vi "Command Drive Distance.vi"(6 "Timeout":dbl=2.0, 8 "Speed":dbl=0.7, 9 "Heading":dbl, 10 "Distance(Feet)":dbl=-8.0, 11 "Startup":bool) -> (0 "Angular":dbl, 1 "Reinit":bool, 2 "Linear":dbl, 3 "Completed":bool=TRUE)   [LabVIEW 2019]
uses:
  Subsystems/Sensing/Sensor_Values.vi
  Auto Utilities/Command_Execution_State.ctl
panel:
  in  "Angle_Threshold":dbl=5.0
  in  "Agressive Turn P":dbl=0.2
  in  "Turn I":dbl=0.0001
  in  "Turn D":dbl=0.005
  out "Turning":cluster{"Heading":dbl, "Drive_IMU":dbl}(graph)={"Heading"=0.0, "Drive_IMU"=0.3076171875}
  in  "Normal Turn P":dbl=0.03
  in  "Distance Gain":dbl=0.01
  # "Alpha .06"
  # "Beta .1"
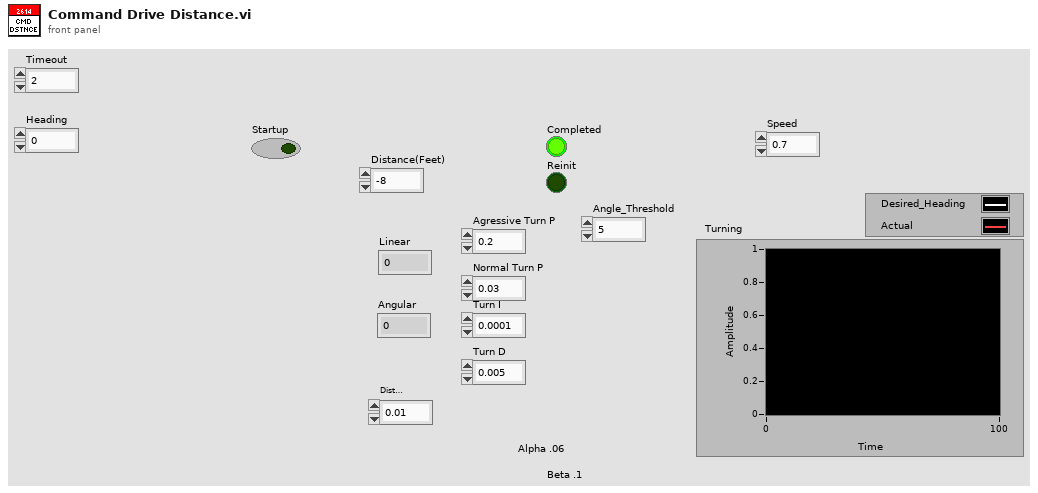
[diagram p1: front panel]
types:
  T1 = typedef "Command_Execution_State.ctl" = enum16{"Initialize", "Execute", "Finish"}
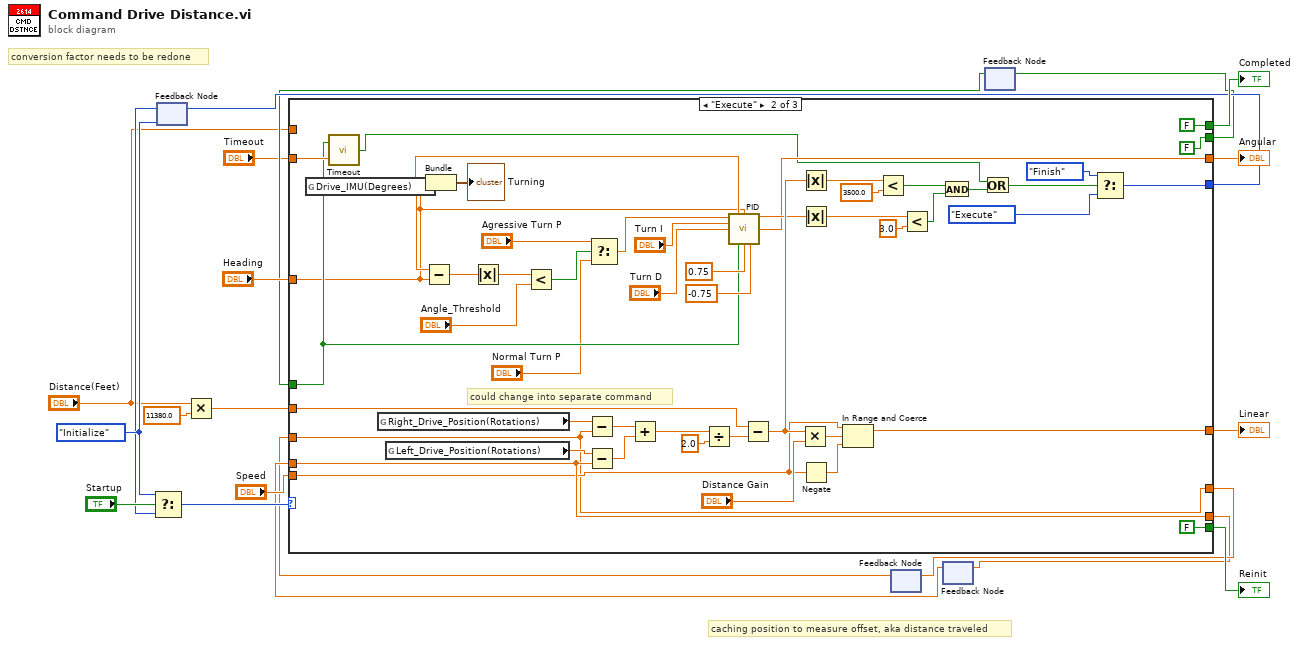
[diagram p0: block diagram]
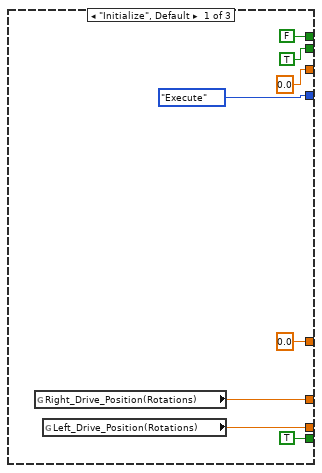
[diagram p2: hidden frame]
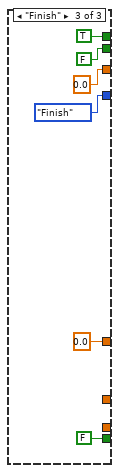
[diagram p3: hidden frame]
diagram:
  w19 = Command_Execution_State."Initialize"
  # "conversion factor needs to be redone"
  # "caching position to measure offset, aka distance traveled"
  n1 = feedback #1(w19) -> (w15:T1)
  n2 = Select(t=w19, s="Startup", f=w15) -> (s? t:f=w20:T1)
  n3 = Multiply(x="Distance(Feet)", y=11380.0) -> (x*y=w5:dbl)
  n4 = feedback #2() -> (w3:dbl)  [unwired: 1 in]
  n5 = feedback #3() -> (w7:dbl)  [unwired: 1 in]
  n6 = feedback #4() -> (w10:bool)  [unwired: 1 in]
  n7 = case shown="\"Execute\"" w20 {
    tunnel: [FALSE FALSE TRUE] -> w18
    tunnel: [TRUE FALSE FALSE] -> w17
    tunnel: [Command_Execution_State."Execute" w75 Command_Execution_State."Finish"] -> w16
    tunnel: [0.0 ("Left Wheel Velocity") w58 0.0] -> w14
    tunnel: [0.0 ("Right Wheel Velocity") w52 0.0] -> w13
    tunnel: "Heading" -> [_ w36 _]
    tunnel: [TRUE FALSE FALSE] -> w11
    tunnel: w10 -> [_ w53 _]
    tunnel: "Timeout" -> [_ w55 _]
    tunnel: "Speed" -> [_ w48 _]
    tunnel: [w22 w30 _] -> w2
    tunnel: [w23 w59 _] -> w1
    tunnel: w3 -> [_ w30 _]
    tunnel: w7 -> [_ w59 _]
    tunnel: w5 -> [_ w47 _]
    tunnel: "Distance(Feet)" -> [_ _ _]
    frame "Initialize", Default {
      n8 = global read "Sensor_Values.vi" "Right_Drive_Position(Rotations)"() -> (w22:dbl)
      n9 = global read "Sensor_Values.vi" "Left_Drive_Position(Rotations)"() -> (w23:dbl)
    }
    frame "Execute" {
      # "could change into separate command"
      n10 = global read "Sensor_Values.vi" "Drive_IMU(Degrees)"() -> (w37:dbl)
      n11 = call "Timeout.vi"("Timeout"=w55, "Initialize"=w53) -> ("Timed Out?"=w44:bool)
      n12 = global read "Sensor_Values.vi" "Right_Drive_Position(Rotations)"() -> (w51:dbl)
      n13 = global read "Sensor_Values.vi" "Left_Drive_Position(Rotations)"() -> (w50:dbl)
      n14 = Subtract(x=w37, y=w36) -> (x-y=w35:dbl)
      n15 = Bundle("Heading"=w36, "Drive_IMU(Degrees)"=w37) -> (→"Turning":cluster{"Heading":dbl, "Drive_IMU(Degrees)":dbl})  [unwired: 1 in]
      n16 = Absolute Value(x=w35) -> (abs(x)=w34:dbl)
      n17 = Less?(x=w34, y="Angle_Threshold") -> (x < y?=w38:bool)
      n18 = Subtract(x=w51, y=w30) -> (x-y=w62:dbl)
      n19 = Subtract(x=w50, y=w59) -> (x-y=w60:dbl)
      n20 = Select(t="Agressive Turn P", s=w38, f="Normal Turn P") -> (s? t:f=w39:dbl)
      n21 = Add(x=w62, y=w60) -> (x+y=w63:dbl)
      n22 = Divide(x=w63, y=2.0) -> (x/y=w64:dbl)
      n23 = call "PID.vi"("Kp"=w39, "Process Variable"=w37, "Goal"=w36, "Ki"="Turn I", "Kd"="Turn D", "Reinit"=w53, "Max Ouput"=0.75, "Min Output"=-0.75) -> ("Current Error"=w54:dbl, "Command"=w52:dbl)  [unwired: 5 in, 1 out]
      n24 = Subtract(x=w47, y=w64) -> (x-y=w73:dbl)
      n25 = Multiply(x=w73, y="Distance Gain") -> (x*y=w71:dbl)
      n26 = Absolute Value(x=w73) -> (abs(x)=w74:dbl)
      n27 = Absolute Value(x=w54) -> (abs(x)=w68:dbl)
      n28 = Negate(x=w48) -> (-x=w49:dbl)
      n29 = In Range and Coerce(upper limit=w48, x=w71, lower limit=w49) -> (coerced(x)=w58:dbl)  [unwired: 1 out]
      n30 = Less?(x=w74, y=3500.0) -> (x < y?=w46:bool)
      n31 = Less?(x=w68, y=3.0) -> (x < y?=w67:bool)
      n32 = And(x=w46, y=w67) -> (x .and. y?=w43:bool)
      n33 = Or(x=w44, y=w43) -> (x .or. y?=w45:bool)
      n34 = Select(t=Command_Execution_State."Finish", s=w45, f=Command_Execution_State."Execute") -> (s? t:f=w75:T1)
    }
    frame "Finish" {
    }
  }
  "Completed" <- w18
  "Reinit" <- w17
  "Linear" <- w14
  "Angular" <- w13
  n35 = feedback-in #1(w16) -> ()
  n36 = feedback-in #2(w2) -> ()
  n37 = feedback-in #3(w1) -> ()
  n38 = feedback-in #4(w11) -> ()
